vi "Keithley 2200 Series Create and Save a List.vi"() -> ()   [LabVIEW 2021]
doc: "DESCRIPTION:\n\nIn this VI commands executed in a certain order to successfully complete a list file. \n\nINSTRUCTIONS:\n1. Enter the resource name.\n2. Set a list in continuous or step mode with command order.\n3. Sets the voltage or current step. \n4. Sets the step time.\n5. Select Save or Recall operation ,to save or recall list file to or from memory \n6. Enter Non -volatile memory address, that the settings will be saved to. \n7. Configures the power supply for command List mode\n8. Run the VI.\n\nNOTES:\n\nNotice the order of the power supply component VIs in the block diagram. The first VI in a sequence is the power supply Initialize.vi, which provides a VISA session to the instrument driver. The last VI in a sequence must be the power supply Close.vi which closes the Visa session."
uses:
  <instrlib>/Keithley 2200 Series/Keithley 2200 Series.lvlib
panel:
  in  "Power Supply Mode (0:Fix)":u16(ring)=1 items=["Fix", "List"]
  in  "Manual Range":dbl[](array[numeric]) format="%.2f"
  in  "Steps Count(2)":dbl=10.0
  in  "Step Time(1)":dbl=1.0
  in  "VISA resource name":refnum<visa-resource-name>
  in  "Memory Address(1)":dbl=1.0
  in  "List Name":string="TEST"
  in  "List Unit(0:Second)":u16(ring) items=["Second", "Msecond"]
  in  "Unit(V)":u16(ring) items=["V", "mV", "A", "mA"]
  in  "List Operation(0:Voltage)":u16(ring) items=["Voltage", "Current"]
  in  "List Repeat Mode(0:Once)":u16(ring) items=["Once", "Repeat  "]
  in  "List Mode(0:Continuous)":u16(ring) items=["Continuous", "Step"]
  # "(c) Copyright 2012 Keithley Instruments Inc  ALL RIGHTS RESERVED."
  # "Configure List Operation"
  # "Configure Mode"
  # "Configure Time"
  # "Save List File"
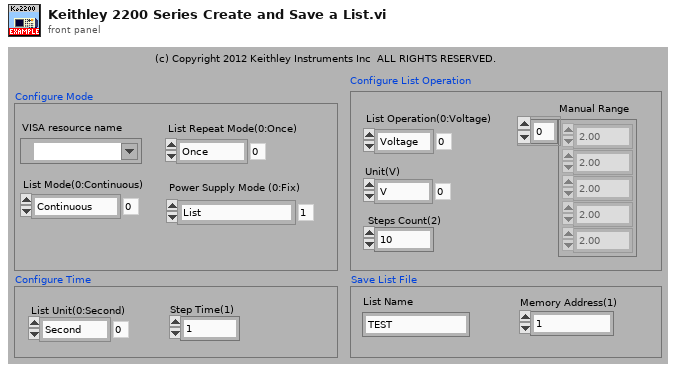
[diagram p1: front panel]
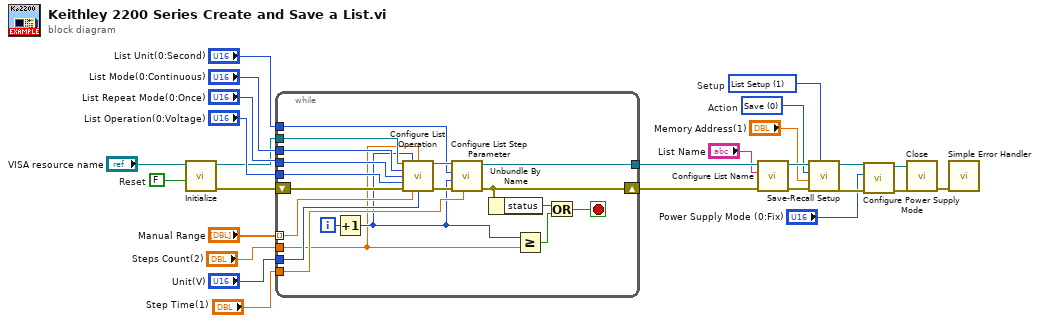
[diagram p0: block diagram]
diagram:
  w1 = u16 1 items=["Instrument Setup", "List Setup"]  # Setup
  w15 = u16 0 items=["Save", "Recall"]  # Action
  w26 = FALSE  # Reset
  n1 = call <instrlib>:"Initialize.vi"("Reset (True)"=w26, "VISA resource name"="VISA resource name") -> ("error out"=w9:errorcluster, "VISA resource name out"=w8:refnum<visa-resource-name>)  [unwired: 3 in, 5 out]
  n2 = while {
    tunnel: "Unit(V)" -> [w45]
    tunnel: [w42] -> w24
    tunnel: "List Mode(0:Continuous)" -> [w41]
    tunnel: "List Repeat Mode(0:Once)" -> [w40]
    tunnel: "List Operation(0:Voltage)" -> [w39]
    tunnel: "List Unit(0:Second)" -> [w38]
    tunnel: "Manual Range" -> [w37] mode=indexing
    tunnel: "Step Time(1)" -> [w36]
    tunnel: "Steps Count(2)" -> [w31]
    tunnel: w8 -> [w34]
    shift-right: [w28] -> w23
    shift-left: w9 -> [w35]
    i -> [w33]
    stop <- w29 stop-if-true
    n3 = Increment(x=w33) -> (x+1=w32:i32)
    n4 = call <instrlib>:"Configure List Operation.vi"("VISA resource name"=w34, "Number of Steps(1)"=w32, "Steps Count(2)"=w31, "List Mode(0:Continuous)"=w41, "List Repeat Mode(0:Once)"=w40, "List Operation(0:Voltage)"=w39, "error in (no error)"=w35, "Manual Range(0.00)"=w37, "Unit(V)"=w45) -> ("VISA resource name out"=w44:refnum<visa-resource-name>, "error out"=w43:errorcluster)  [unwired: 5 out]
    n5 = call <instrlib>:"Configure List Step Parameter.vi"("Step Time(1)"=w36, "error in (no error)"=w43, "List Step Number(2)"=w32, "Unit(S)"=w38, "VISA resource name"=w44) -> ("error out"=w28:errorcluster, "VISA resource name out"=w42:refnum<visa-resource-name>)  [unwired: 5 out]
    n6 = Unbundle By Name(w28) -> ("status"=w27:bool)
    n7 = Greater Or Equal?(x=w32, y=w31) -> (x >= y?=w30:bool)
    n8 = Or(x=w27, y=w30) -> (x .or. y?=w29:bool)
  }
  n9 = call <instrlib>:"Configure List Name.vi"("error in (no error)"=w23, "List Name"="List Name", "VISA resource name"=w24) -> ("error out"=w21:errorcluster, "VISA resource name out"=w22:refnum<visa-resource-name>)  [unwired: 7 out]
  n10 = call <instrlib>:"Save-Recall Setup.vi"("Setup(0:Instrument Setup)"=w1, "error in (no error)"=w21, "Memory Address(1)"="Memory Address(1)", "Action(0:Save)"=w15, "VISA resource name"=w22) -> ("error out"=w5:errorcluster, "VISA resource name out"=w4:refnum<visa-resource-name>)  [unwired: 5 out]
  n11 = call <instrlib>:"Configure Power Supply Mode.vi"("error in (no error)"=w5, "Power Supply Mode (0:Fix)"="Power Supply Mode (0:Fix)", "VISA resource name"=w4) -> ("error out"=w6:errorcluster, "VISA resource name out"=w3:refnum<visa-resource-name>)  [unwired: 7 out]
  n12 = call <instrlib>:"Close.vi"("error in (no error)"=w6, "VISA resource name"=w3) -> ("error out"=w12:errorcluster)  [unwired: 9 out]
  n13 = call <vilib>:"Simple Error Handler.vi"("error in (no error)"=w12) -> ()  [unwired: 1 in, 8 out]
